vi "Write On Board Memory (NVM).vi"(0 "Session Handle in":T1, 1 "Reverse?":bool, 5 "Address":u16=171 format="%x", 7 "Bytes to Write":u8[](array[numeric]), 11 "error in (no error)":errorcluster) -> (4 "Session Handle out":T1, 15 "error out":errorcluster)   [LabVIEW 2015, in "PAS.lvclass"]
uses:
  PAS.lvclass
  Typedefs/Session Handle.ctl
panel:
  out "Whole Payload":u8[](array[numeric])
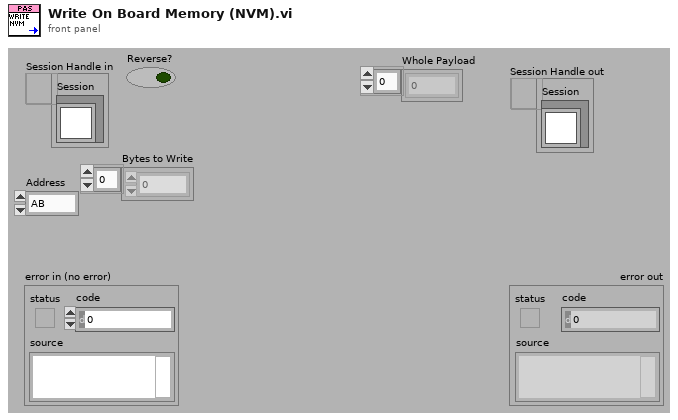
[diagram p1: front panel]
types:
  T1 = typedef "PAS.lvclass/Session Handle.ctl" = refnum<data-value>
  T2 = typedef "XNET Frame CAN.ctl" = cluster{"timestamp":timestamp, "payload":u8[], "identifier":u32, "type":T3, "extended?":bool, "echo?":bool}
  T3 = typedef "XNET Frame Type CAN.ctl" = u8
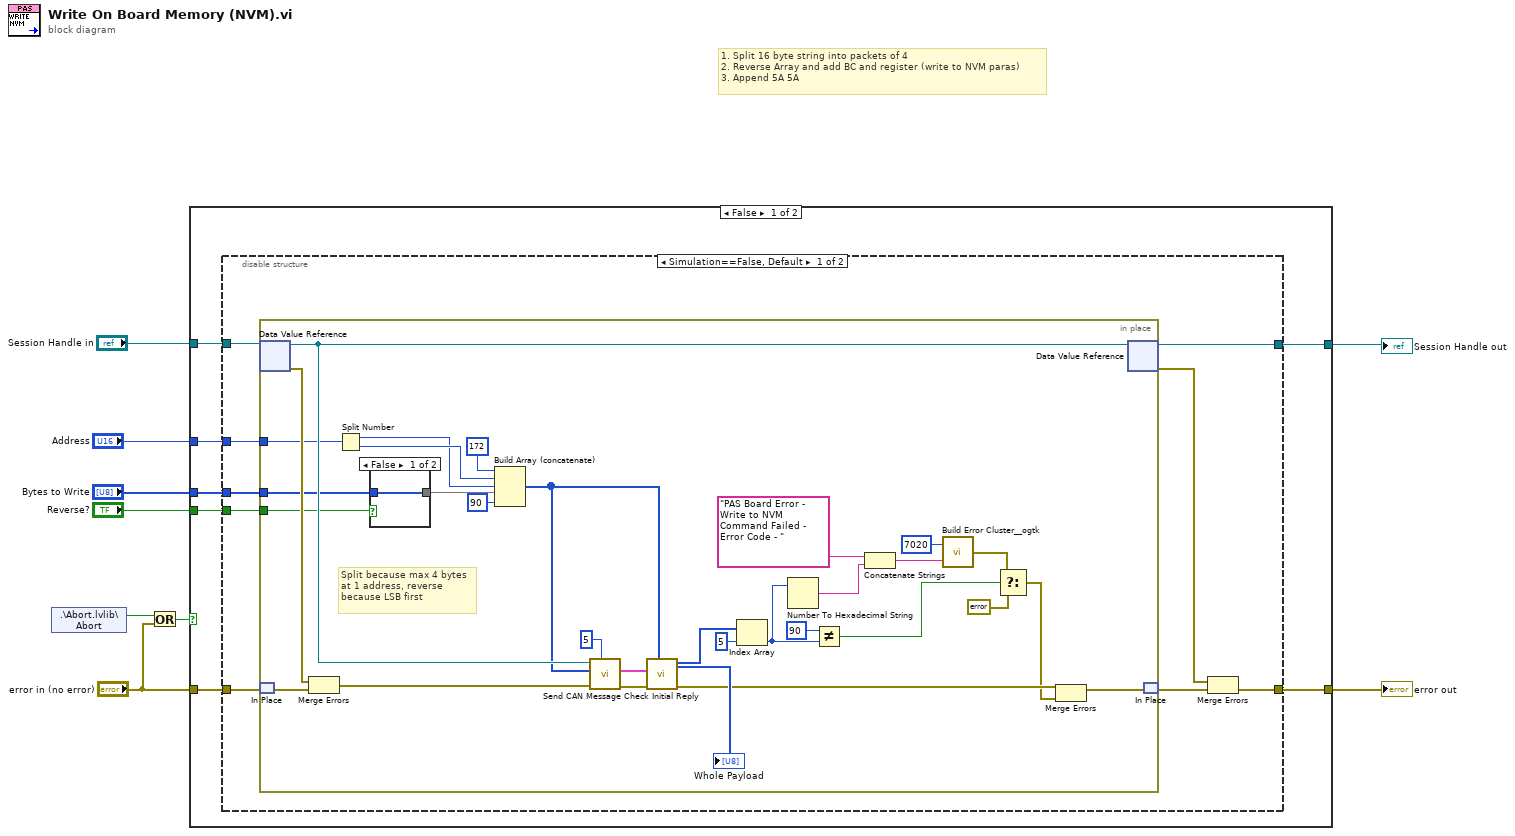
[diagram p0: block diagram]
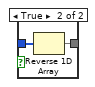
[diagram p2: hidden frame]
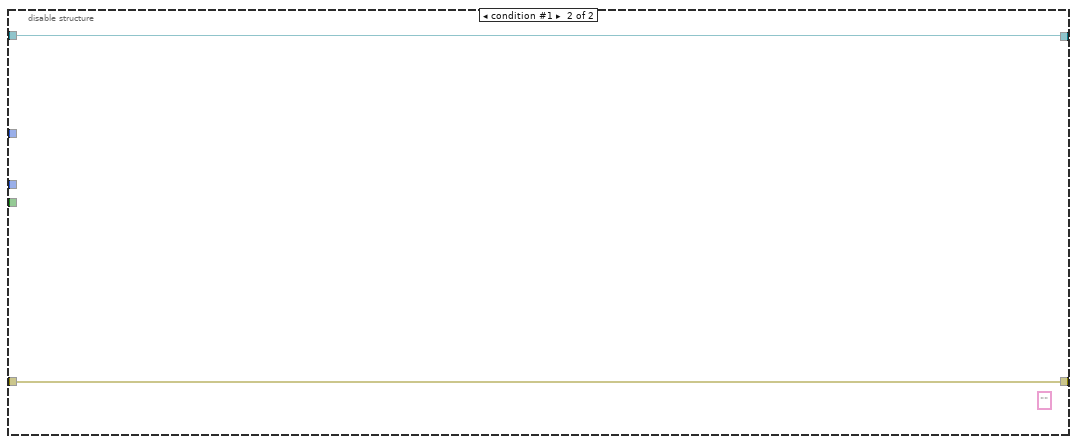
[diagram p3: hidden frame]
diagram:
  # "1. Split 16 byte string into packets of 4\n2. Reverse Array and add BC and register (write to NVM paras)\n3. Append 5A 5A"
  n1 = shared-variable ".\\Abort.lvlib\\Abort"() -> (w6:bool)  [unwired: 1 in, 1 out]
  n2 = Or(x=w6, y="error in (no error)") -> (x .or. y?=w4:bool)
  n3 = case shown="False" w4 {
    tunnel: [w16 w63] -> w8
    tunnel: [w15 w62] -> w7
    tunnel: "Session Handle in" -> [w14 w63]
    tunnel: "error in (no error)" -> [w13 w62]
    tunnel: "Address" -> [w12 _]
    tunnel: "Bytes to Write" -> [w11 _]
    tunnel: "Reverse?" -> [w10 _]
    frame False {
      n4 = disable-structure shown="Simulation==False, Default" {
        disable-tunnel: [w25 w61] -> w16
        disable-tunnel: [w22 w60] -> w15
        disable-tunnel: w14 -> [w21 w61]
        disable-tunnel: w13 -> [w20 w60]
        disable-tunnel: w12 -> [w19 _]
        disable-tunnel: w11 -> [w18 _]
        disable-tunnel: w10 -> [w17 _]
        frame condition #0 (active) {
          n5 = in-place {
            in-place-border: w19 -> [w44]
            in-place-border: w18 -> [w27]
            in-place-border: w17 -> [w26]
            # "Split because max 4 bytes\nat 1 address, reverse \nbecause LSB first"
            n6 = in-place-dvr #1(w21) -> (w53:refnum<class "PAS.lvclass">, w56:errorcluster)
            n7 = in-place-match #2(w20) -> (w55:errorcluster)
            n8 = Merge Errors(w56, w55) -> (w54:errorcluster)
            n9 = Split Number(x=w44) -> (hi(x)=w42:u8, lo(x)=w43:u8)
            n10 = case shown="False" w26 {
              tunnel: [w57 w59] -> w32
              tunnel: w27 -> [w57 w58]
              frame False {
              }
              frame True {
                n11 = Reverse 1D Array(array=w58) -> (reversed array=w59:u8[])
              }
            }
            n12 = Build Array (concatenate)(u8 172, w43, w42, w32, u8 90) -> (w48:u8[])
            n13 = call "Send CAN Message.vi"("Number of Retries"=5, "error in (no error)"=w54, "payload"=w48, "Gas In"=w53) -> ("error out"=w30:errorcluster, "Reply"=w49:T2[])  [unwired: 5 in, 1 out]
            n14 = call "Check Initial Reply.vi"("Write Message"=w48, "error in (no error)"=w30, "Reply"=w49) -> ("error out"=w29:errorcluster, "Data Packet"=w41:u8[], "Whole Payload"=→"Whole Payload":u8[])  [unwired: 5 in, 1 out]
            n15 = Index Array(array=w41, index=5) -> (element=w37:u8)
            n16 = Number To Hexadecimal String(2:w37) -> (0:w36:string)  [unwired: 1 in]
            n17 = Not Equal?(x=u8 90, y=w37) -> (x != y?=w34:bool)
            n18 = Concatenate Strings("PAS Board Error - Write to NVM Command Failed - Error Code - " ("string"), w36) -> (w35:string)
            n19 = call <userlib>:"Build Error Cluster__ogtk.vi"("String to Prepend to source (\"\")"=w35, "code"=7020) -> ("error out"=w46:errorcluster)
            n20 = Select(t=w46, s=w34, f=errorcluster {"status"=FALSE, "code"=0, "source"=""}) -> (s? t:f=w28:errorcluster)
            n21 = Merge Errors(w29, w28) -> (w52:errorcluster)
            n22 = in-place-dvr #1(w53) -> (w25:T1, w23:errorcluster)
            n23 = in-place-match #2(w52) -> (w24:errorcluster)
          }
          n24 = Merge Errors(w23, w24) -> (w22:errorcluster)
        }
        frame condition #1 {
          (unwired) "" ("string")
        }
      }
    }
    frame True {
    }
  }
  "Session Handle out" <- w8
  "error out" <- w7
